vi "Max and Min.vi"() -> ()   [LabVIEW 2023]
doc: "This example shows how the Max & Min function operates with different data types."
panel:
  in  "Tab Control":T1(tab)
  out "Max of X and Y":i32
  out "Min of X and Y":i32
  in  "Numeric Y":i32=56
  in  "Numeric X":i32=45
  out "Min String":string
  out "Max String":string
  in  "String Y":string="test ABC"
  in  "String X":string="test D"
  out "Min Path":path
  out "Max Path":path
  in  "Path Y":path=path "C:/Test1234"
  in  "Path X":path=path "C:/Test2"
  out "Maximum Cluster":T2
  out "Minimum Cluster":T2
  in  "Input Cluster Y":T2={"Numeric"=0.0, "String"="VI", "Numeric 2"=7.0}
  in  "Input Cluster X":T2={"Numeric"=1.0, "String"="test", "Numeric 2"=-3.0}
  out "Earliest Time":timestamp
  out "Latest Time":timestamp
  in  "Time Stamp Y":timestamp=timestamp(2327499010.485 s since 1904-01-01)
  in  "Time Stamp X":timestamp=timestamp(3084908797.174 s since 1904-01-01)
  out "Min Array":dbl[](array[numeric])
  out "Max Array":dbl[](array[numeric])
  in  "Array Y":dbl[](array[numeric])=[1.0, 2.0, 3.0, 4.0]
  in  "Array X":dbl[](array[numeric])=[5.0, 4.0, 3.0, 2.0, 1.0]
  # "Overview: Demonstrates how the Max & Min function operates with different data types.\nInstructions:\n1. Run the VI.\n2. Examine the different cases."
  # "Max & Min finds the maximum and minimum of two numeric values."
  # "Max & Min compares the two strings character by character until it finds a character that has a higher ASCII numeric value. String length is not taken into account."
  # "Max & Min compares the two paths character by character until it finds a character that has a higher ASCII numeric value. Path length is not taken into account."
  # "Max & Min compares the clusters element by element, and returns clusters of the comparison results. The resulting clusters will have the same data type as the input clusters."
  # "Max & Min finds the latest time (maximum) and earliest time (minimum) of two time stamp values."
  # "Max & Min compares the arrays element by element, and returns arrays of the comparison results. The resulting arrays will be the same size as the smaller of the two input arrays."
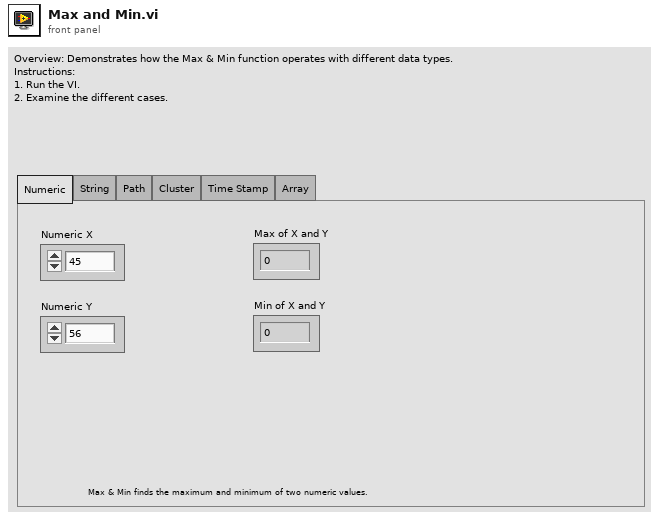
[diagram p1: front panel]
types:
  T1 = enum32{"Numeric", "String", "Path", "Cluster", "Time Stamp", "Array"}
  T2 = cluster{"Numeric":dbl, "String":string, "Numeric 2":dbl}
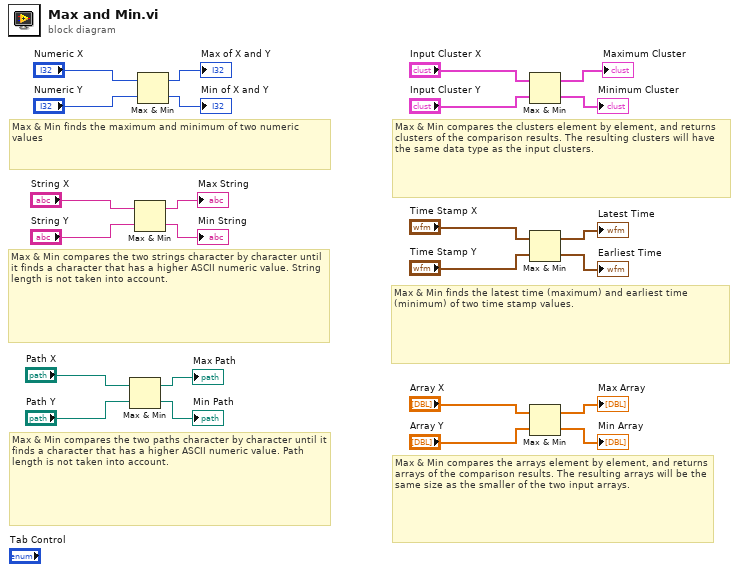
[diagram p0: block diagram]
diagram:
  # "Max & Min finds the latest time (maximum) and earliest time (minimum) of two time stamp values."
  # "Max & Min compares the clusters element by element, and returns clusters of the comparison results. The resulting clusters will have the same data type as the input clusters."
  # "Max & Min compares the two paths character by character until it finds a character that has a higher ASCII numeric value. Path length is not taken into account."
  # "Max & Min compares the two strings character by character until it finds a character that has a higher ASCII numeric value. String length is not taken into account."
  # "Max & Min compares the arrays element by element, and returns arrays of the comparison results. The resulting arrays will be the same size as the smaller of the two input arrays."
  # "Max & Min finds the maximum and minimum of two numeric values"
  n1 = Max & Min(x="Path X", y="Path Y") -> (max(x,y)=→"Max Path":path, min(x,y)=→"Min Path":path)
  n2 = Max & Min(x="String X", y="String Y") -> (max(x,y)=→"Max String":string, min(x,y)=→"Min String":string)
  n3 = Max & Min(x="Numeric X", y="Numeric Y") -> (max(x,y)=→"Max of X and Y":i32, min(x,y)=→"Min of X and Y":i32)
  n4 = Max & Min(x="Input Cluster X", y="Input Cluster Y") -> (max(x,y)=→"Maximum Cluster":T2, min(x,y)=→"Minimum Cluster":T2)
  n5 = Max & Min(x="Time Stamp X", y="Time Stamp Y") -> (max(x,y)=→"Latest Time":timestamp, min(x,y)=→"Earliest Time":timestamp)
  n6 = Max & Min(x="Array X", y="Array Y") -> (max(x,y)=→"Max Array":dbl[], min(x,y)=→"Min Array":dbl[])
